vi "average_exp_simpleSD.vi"(2 "Name cluster":cluster{"Name":string, "Comments":string}, 3 "cluster in":T1={"Kinetics"=[], "Spectrum"=[], "Experiments groups"=[], "GRAPH EXPERIMENTAL DATA"=[], "error out"={"status"=FALSE, "code"=0, "source"=""}, "group"=0, "exp selected"=0, "# exp"=0, "kinetics plot names"=[], "spectra plot names"=[], "FromToWave"={"FromWave"=0.0, "ToWave"=0.0}, "Laser shutter task"="", "Accelerator task"="", "Motor task"="", "GRAPH EXPERIMENTAL DATA ref"=refnum, "timedelays"=[0.0, 0.0, 0.0, 0.0, 0.0, 0.0, 0.0, 0.06019061100911815, 0.0521779104562645, 0.045231877429679615, 0.03921051490799832, 0.033990728811568754, 0.029465811603150715, 0.025543260876973825, 0.02214288834180205, 0.01919518054014414, 0.016639877791965713, 0.014424742312398925, 0.012504490320209958, 0.010839866306230088, 0.009396840537117498, 0.008145913389103785, 0.00706151229029317, 0.006121468943269439, 0.005306566140927374, 0.004600144911132549, 0.003987763959109073, 0.0034569044455719407, 0.00299671406541447, 0.0025977851951783253, 0.0022519625739982996, 0.00195217658646366, 0.0016922987392150965, 0.0014670163768006634, 0.0012717240756200802, 0.0011024294957352762, 0.0009556717658856477, 0.0008284507332614981, 0.0007181656316962257, 0.0006225619144775864, 0.0005396851648867825, 0.00046784114226338394, 0.0004055611468220084, 0.0003515719951773376, 0.00030476999279031153, 0.00026419837125694315, 0.00022902772919263772, 0.0001985390768670671, 0.0001721091379728629, 0.00014919760805372974, 0.00012933610911736794], "wavelengths"=[0.0, 0.0, 0.0, 0.0, 0.0, 0.0, 0.0, 0.06019061100911815, 0.0521779104562645, 0.045231877429679615, 0.03921051490799832, 0.033990728811568754, 0.029465811603150715, 0.025543260876973825, 0.02214288834180205, 0.01919518054014414, 0.016639877791965713, 0.014424742312398925, 0.012504490320209958, 0.010839866306230088, 0.009396840537117498, 0.008145913389103785, 0.00706151229029317, 0.006121468943269439, 0.005306566140927374, 0.004600144911132549, 0.003987763959109073, 0.0034569044455719407, 0.00299671406541447, 0.0025977851951783253, 0.0022519625739982996, 0.00195217658646366, 0.0016922987392150965, 0.0014670163768006634, 0.0012717240756200802, 0.0011024294957352762, 0.0009556717658856477, 0.0008284507332614981, 0.0007181656316962257, 0.0006225619144775864, 0.0005396851648867825, 0.00046784114226338394, 0.0004055611468220084, 0.0003515719951773376, 0.00030476999279031153, 0.00026419837125694315, 0.00022902772919263772, 0.0001985390768670671, 0.0001721091379728629, 0.00014919760805372974, 0.00012933610911736794], "Experiment"=refnum, "Commentaires exp"=refnum, "FromToDelay"={"FromDelay"=0.0, "ToDelay"=0.0}}) -> (0 "cluster out":T1={"Kinetics"=[], "Spectrum"=[], "Experiments groups"=[], "GRAPH EXPERIMENTAL DATA"=[], "error out"={"status"=FALSE, "code"=0, "source"=""}, "group"=0, "exp selected"=0, "# exp"=0, "kinetics plot names"=[], "spectra plot names"=[], "FromToWave"={"FromWave"=0.0, "ToWave"=0.0}, "Laser shutter task"="", "Accelerator task"="", "Motor task"="", "GRAPH EXPERIMENTAL DATA ref"=refnum, "timedelays"=[0.0, 0.0, 0.0, 0.0, 0.0, 0.0, 0.0, 0.06019061100911815, 0.0521779104562645, 0.045231877429679615, 0.03921051490799832, 0.033990728811568754, 0.029465811603150715, 0.025543260876973825, 0.02214288834180205, 0.01919518054014414, 0.016639877791965713, 0.014424742312398925, 0.012504490320209958, 0.010839866306230088, 0.009396840537117498, 0.008145913389103785, 0.00706151229029317, 0.006121468943269439, 0.005306566140927374, 0.004600144911132549, 0.003987763959109073, 0.0034569044455719407, 0.00299671406541447, 0.0025977851951783253, 0.0022519625739982996, 0.00195217658646366, 0.0016922987392150965, 0.0014670163768006634, 0.0012717240756200802, 0.0011024294957352762, 0.0009556717658856477, 0.0008284507332614981, 0.0007181656316962257, 0.0006225619144775864, 0.0005396851648867825, 0.00046784114226338394, 0.0004055611468220084, 0.0003515719951773376, 0.00030476999279031153, 0.00026419837125694315, 0.00022902772919263772, 0.0001985390768670671, 0.0001721091379728629, 0.00014919760805372974, 0.00012933610911736794], "wavelengths"=[0.0, 0.0, 0.0, 0.0, 0.0, 0.0, 0.0, 0.06019061100911815, 0.0521779104562645, 0.045231877429679615, 0.03921051490799832, 0.033990728811568754, 0.029465811603150715, 0.025543260876973825, 0.02214288834180205, 0.01919518054014414, 0.016639877791965713, 0.014424742312398925, 0.012504490320209958, 0.010839866306230088, 0.009396840537117498, 0.008145913389103785, 0.00706151229029317, 0.006121468943269439, 0.005306566140927374, 0.004600144911132549, 0.003987763959109073, 0.0034569044455719407, 0.00299671406541447, 0.0025977851951783253, 0.0022519625739982996, 0.00195217658646366, 0.0016922987392150965, 0.0014670163768006634, 0.0012717240756200802, 0.0011024294957352762, 0.0009556717658856477, 0.0008284507332614981, 0.0007181656316962257, 0.0006225619144775864, 0.0005396851648867825, 0.00046784114226338394, 0.0004055611468220084, 0.0003515719951773376, 0.00030476999279031153, 0.00026419837125694315, 0.00022902772919263772, 0.0001985390768670671, 0.0001721091379728629, 0.00014919760805372974, 0.00012933610911736794], "Experiment"=refnum, "Commentaires exp"=refnum, "FromToDelay"={"FromDelay"=0.0, "ToDelay"=0.0}}, 1 "Exp Avg Name":string)   [LabVIEW 2015]
uses:
  controls/control-cluster.ctl
  Classes/Experiments_group.lvclass
  Classes/Experiment.lvclass
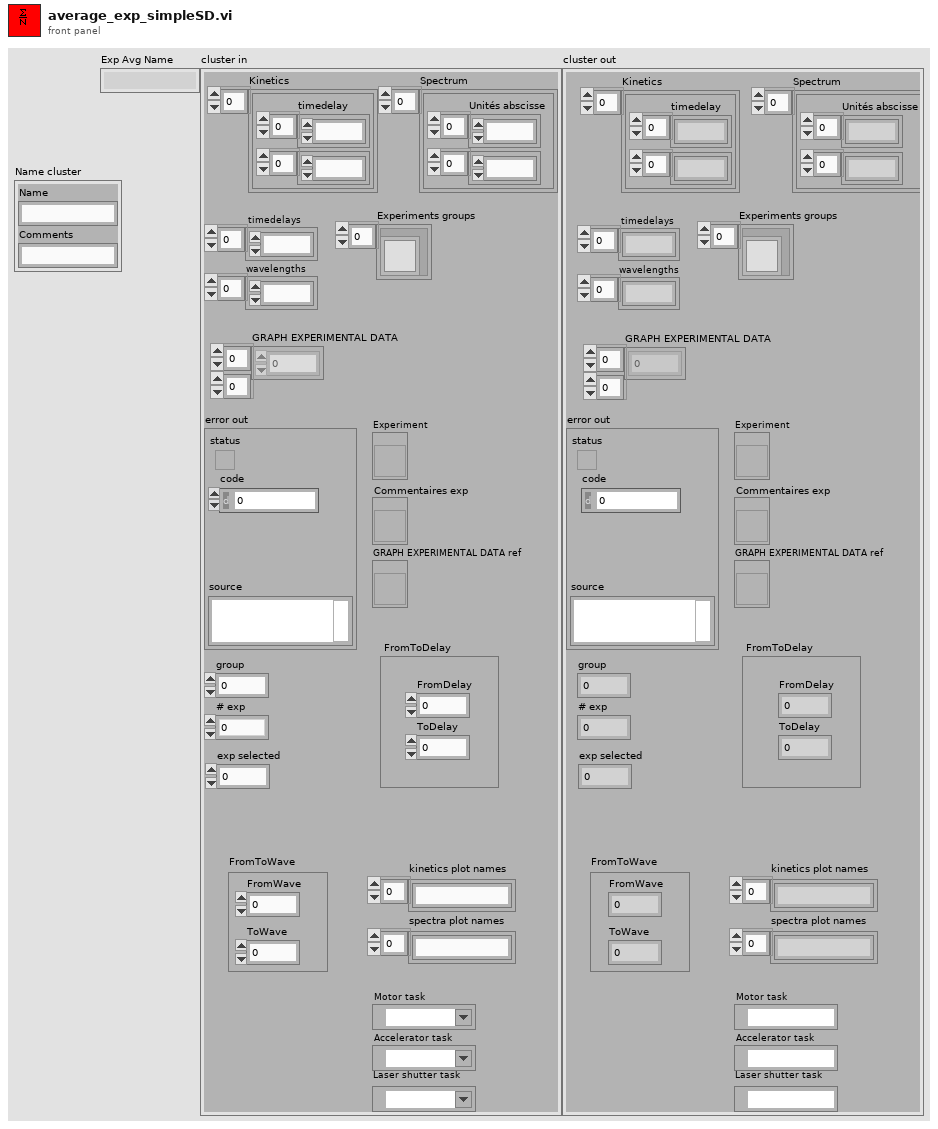
[diagram p1: front panel]
types:
  T1 = typedef "control-cluster.ctl" = cluster{"Kinetics":cluster{"timedelay":dbl[], dbl[]}[], "Spectrum":cluster{"Unités abscisse":dbl[], dbl[]}[], "Experiments groups":refnum<class "Experiments_group.lvclass">[], "GRAPH EXPERIMENTAL DATA":dbl[][], "error out":errorcluster, "group":i32, "exp selected":i32, "# exp":i32, "kinetics plot names":string[], "spectra plot names":string[], "FromToWave":cluster{"FromWave":dbl, "ToWave":dbl}, "Laser shutter task":refnum<k21>, "Accelerator task":refnum<k21>, "Motor task":refnum<k21>, "GRAPH EXPERIMENTAL DATA ref":refnum<vi>, "timedelays":dbl[], "wavelengths":dbl[], "Experiment":refnum<vi>, "Commentaires exp":refnum<vi>, "FromToDelay":cluster{"FromDelay":dbl, "ToDelay":dbl}}
  T2 = typedef "mylistbox.ctl" = i32[]
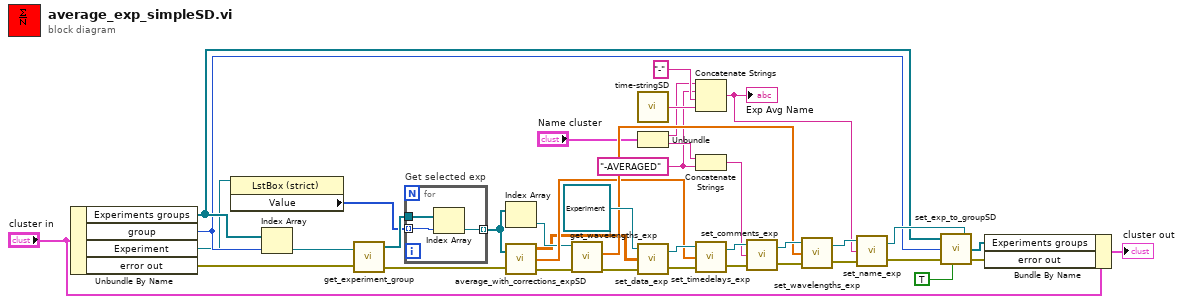
[diagram p0: block diagram]
diagram:
  w16 = "-AVERAGED" ("string")
  n1 = Unbundle By Name("cluster in") -> ("Experiments groups"=w9:refnum<class "Experiments_group.lvclass">[], "group"=w8:i32, "Experiment"=w7:refnum<vi>, "error out"=w6:errorcluster)
  n2 = property class="LstBox (strict)"(reference=w7) -> ("Value"=w37:T2)  [unwired: 1 in, 2 out]
  n3 = Index Array(array=w9, index=w8) -> (element=w39:refnum<class "Experiments_group.lvclass">)
  n4 = call-dynamic "get_experiment_group.vi"("Experiments_group.lvclass in"=w39, "error in (no error)"=w6) -> ("Experiments"=w38:refnum<class "Experiment.lvclass">[], "error out"=w10:errorcluster)  [unwired: 1 out]
  n5 = for "Get selected exp" {
    tunnel: w38 -> [w42]
    tunnel: w37 -> [w41] mode=indexing
    tunnel: [w40] -> w36 mode=indexing
    n6 = Index Array(array=w42, index=w41) -> (element=w40:refnum<class "Experiment.lvclass">)
  }
  n7 = Index Array(array=w36) -> (element=w14:refnum<class "Experiment.lvclass">)  [unwired: 1 in]
  n8 = call "average_with_corrections_expSD.vi"("all exp to average"=w36, "error in (no error)"=w10) -> ("averaged without bad points"=w13:dbl[][], "timedelays longest"=w15:dbl[], "sortie d'erreur"=w12:errorcluster)
  n9 = call-dynamic "get_wavelengths_exp.vi"("error in (no error)"=w12, "Experiment.lvclass in"=w14) -> ("error out"=w11:errorcluster, "wavelengths"=w23:dbl[])  [unwired: 7 in, 1 out]
  n10 = call "time-stringSD.vi"() -> ("time"=w18:string)
  n11 = Unbundle("Name cluster") -> ("Name"=w17:string, "Comments"=w20:string)
  n12 = call-dynamic "set_data_exp.vi"("error in (no error)"=w11, "Data"=w13, "Experiment.lvclass in"=refnum<class "Experiment.lvclass"> refnum) -> ("error out"=w30:errorcluster, "Experiment.lvclass out"=w34:refnum<class "Experiment.lvclass">)
  n13 = Concatenate Strings(w17, w16, "-" ("string"), w18) -> (w1:string)
  "Exp Avg Name" <- w1
  n14 = Concatenate Strings(w20, w16) -> (w22:string)
  n15 = call-dynamic "set_timedelays_exp.vi"("error in (no error)"=w30, "timedelays"=w15, "Experiment.lvclass in"=w34) -> ("error out"=w29:errorcluster, "Experiment.lvclass out"=w33:refnum<class "Experiment.lvclass">)
  n16 = call-dynamic "set_comments_exp.vi"("error in (no error)"=w29, "Comments"=w22, "Experiment.lvclass in"=w33) -> ("error out"=w28:errorcluster, "Experiment.lvclass out"=w32:refnum<class "Experiment.lvclass">)
  n17 = call-dynamic "set_wavelengths_exp.vi"("error in (no error)"=w28, "wavelengths"=w23, "Experiment.lvclass in"=w32) -> ("error out"=w27:errorcluster, "Experiment.lvclass out"=w31:refnum<class "Experiment.lvclass">)
  n18 = call-dynamic "set_name_exp.vi"("error in (no error)"=w27, "Exp name"=w1, "Experiment.lvclass in"=w31) -> ("error out"=w24:errorcluster, "Experiment.lvclass out"=w25:refnum<class "Experiment.lvclass">)
  n19 = call "set_exp_to_groupSD.vi"("Experiments groups"=w9, "group"=w8, "error in (no error)"=w24, "New"=TRUE, "Experiment in"=w25) -> ("Experiments groups out"=w4:refnum<class "Experiments_group.lvclass">[], "error out"=w2:errorcluster)  [unwired: 1 in]
  n20 = Bundle By Name(cluster="cluster in", "Experiments groups"=w4, "error out"=w2) -> (→"cluster out":T1)
